vi "Convert Surface.vi"(6 "Flags":u32 format="%.0x", 8 "error in":errorcluster, 10 "Pixel Format Pointer":u32 format="%.0x", 11 "Loaded Surface Pointer":u32 format="%.0x") -> (0 "error out":errorcluster, 3 "Surface Pointer":u32 format="%.0x")   [LabVIEW 2014, in "LibSDL2.lvlib"]
uses:
  LibSDL2.lvlib
  DLL/SDL2.dll
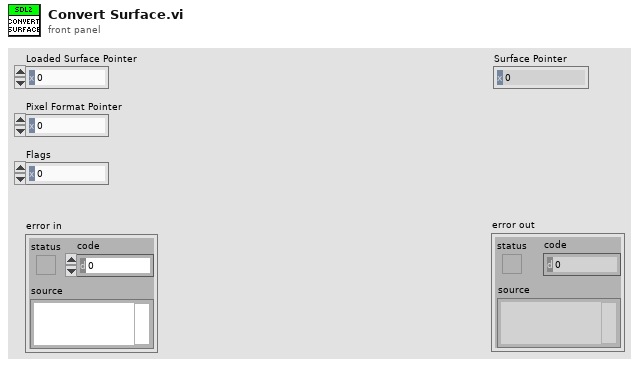
[diagram p1: front panel]
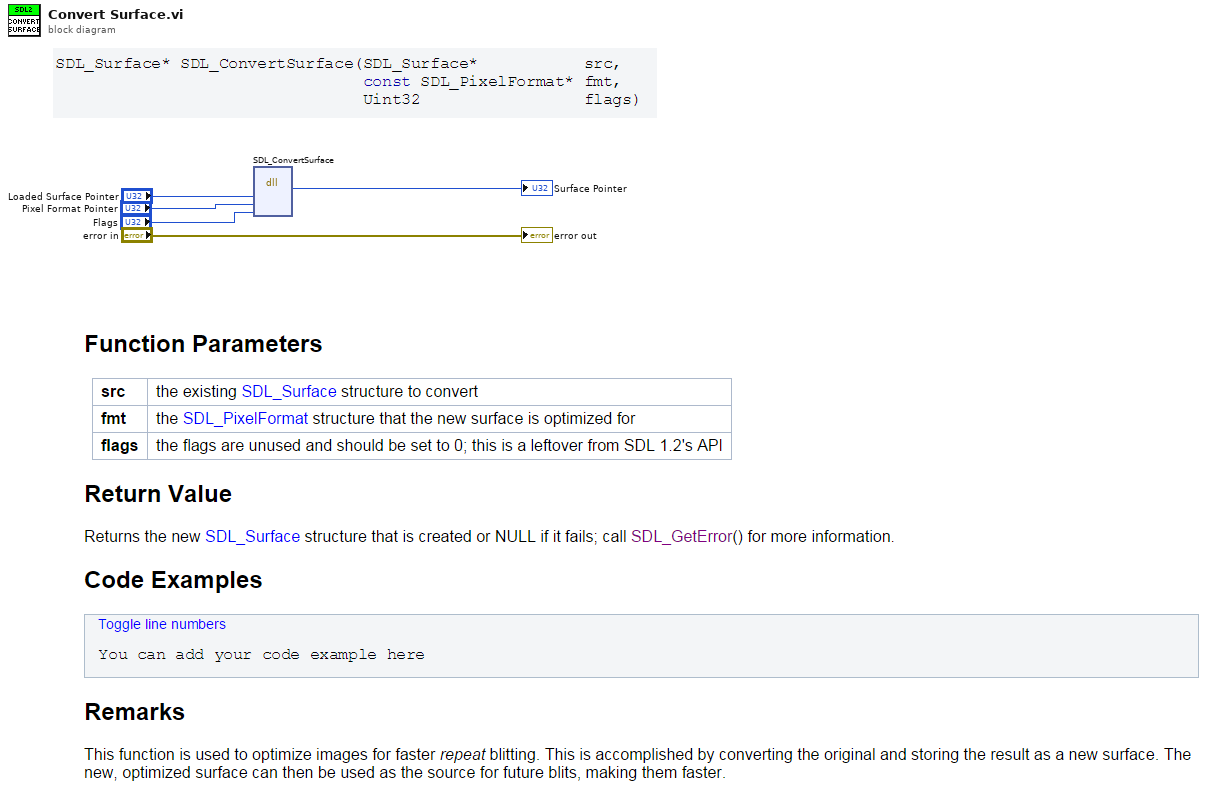
[diagram p0: block diagram]
diagram:
  n1 = dll-call lib="C:/dev/PGS/LabSDL2/Source/LibSDL2 Wrapper/DLL/SDL2.dll" fn="SDL_ConvertSurface"("src"="Loaded Surface Pointer", "fmt"="Pixel Format Pointer", "flags"="Flags") -> ("surface pointer"=→"Surface Pointer":u32)  [unwired: 6 in, 2 out]
  "error out" <- "error in"
